vi "Add Linked List.vi"(6 "Insertion Index":i32=-1, 7 "Parent ID":string, 8 "error in (no error)":errorcluster, 9 "Linked List ID":string, 10 "Name":string, 11 "ILinked List in":refnum<class "ILinked List.lvclass">) -> (0 "error out":errorcluster, 1 "Replaced?":bool, 3 "ILinked List out":refnum<class "ILinked List.lvclass">, 5 "Unique ID out":string)   [LabVIEW 2017, in "Linked Lists.lvlib" / "ILinked List.lvclass"]
uses:
  <vilib>/gpm_packages/@cs/linked-list/Source/Linked List/ILinkedList/ILinked List.lvclass
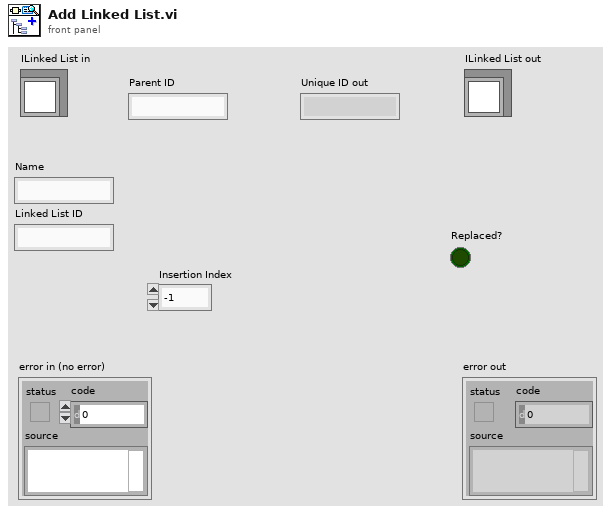
[diagram p1: front panel]
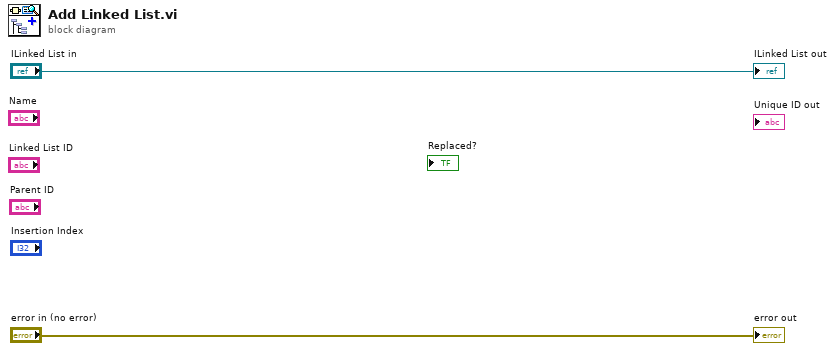
[diagram p0: block diagram]
diagram:
  "error out" <- "error in (no error)"
  "ILinked List out" <- "ILinked List in"
